vi "Populate Module.vi"(4 "Manifestation Ancestors":T1, 7 "Temporary Template Root Dir":path, 9 "Preloaded Module Class Ref Map":variant, 10 "Module Spec. File":path, 11 "Module LVLib":refnum<vi>) -> (3 "Module LVLib Dup":refnum<vi>)   [LabVIEW 2013]
doc: "Copyright (c) 2016 Sze Howe Koh\n\nThis Source Code Form is subject to the terms of the Mozilla Public License, v. 2.0. If a copy of the MPL was not distributed with this file, You can obtain one at http://mozilla.org/MPL/2.0/."
uses:
  Data Structures/Manifestation Ancestors.ctl
  Param Writers/TypeConv/Category.ctl
  Param Writers/Identity Writer/Identity Writer.lvclass
  Param Writers/Opaque Struct Writer/Opaque Struct Writer.lvclass
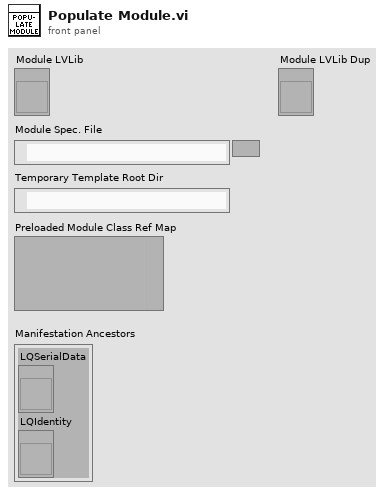
[diagram p1: front panel]
types:
  T1 = typedef "Manifestation Ancestors.ctl" = cluster{"LQSerialData":refnum<vi>, "LQIdentity":refnum<vi>}
  T2 = typedef "Category.ctl" = enum16{"Invalid", "Void", "Boolean", "Numeric", "Enum", "SimpleStruct", "OpaqueStruct", "SimpleIdentity", "QObject", "SimpleContainer", "FullArray"}
  T3 = typedef "Type Categories.ctl" = cluster{"numerics":T4[], "simpleStructs":T5[], "opaqueStructs":T10[], "simpleIdentities":T10[], "qObjects":T10[], "simpleContainers":T4[], "fullArrays":T4[]}
  T4 = typedef "TypeConv.ctl" = cluster{"name":string, "dllType":string}
  T5 = typedef "Simple Struct.ctl" = cluster{"name":string, "fields":T6[], "methods":T7[]}
  T6 = typedef "Param.ctl" = cluster{"name":string, "type":string, "defaultValue":string}
  T7 = typedef "Method.ctl" = cluster{"name":string, "retType":string, "uniqueName":string, "params":T6[], "isConst":bool, "isStaticMember":bool, "isFactory":bool, "connectorPane":T8}
  T8 = typedef "Connector Pane.ctl" = cluster{"pattern":u32, "terminals":T9[]}
  T9 = typedef "Connector Pane Terminal.ctl" = cluster{"name":string, "index":u32}
  T10 = typedef "Class.ctl" = cluster{"name":string, "base":string, "enums":T11[], "methods":T7[], "properties":T13[]}
  T11 = typedef "Enum.ctl" = cluster{"name":string, "values":T12[]}
  T12 = typedef "Enum Value.ctl" = cluster{"name":string, "value":i32}
  T13 = typedef "Property.ctl" = cluster{"name":string, "getter":string, "setter":string}
  T14 = typedef "Namespace.ctl" = cluster{"name":string, "enums":T11[], "methods":T7[]}
  T15 = typedef "Projection Info.ctl" = cluster{"source":string, "projection":string}
  T16 = typedef "LabVIEW Documentation.ctl" = cluster{"classUrlFormat":string, "methodUrlFormat":string}
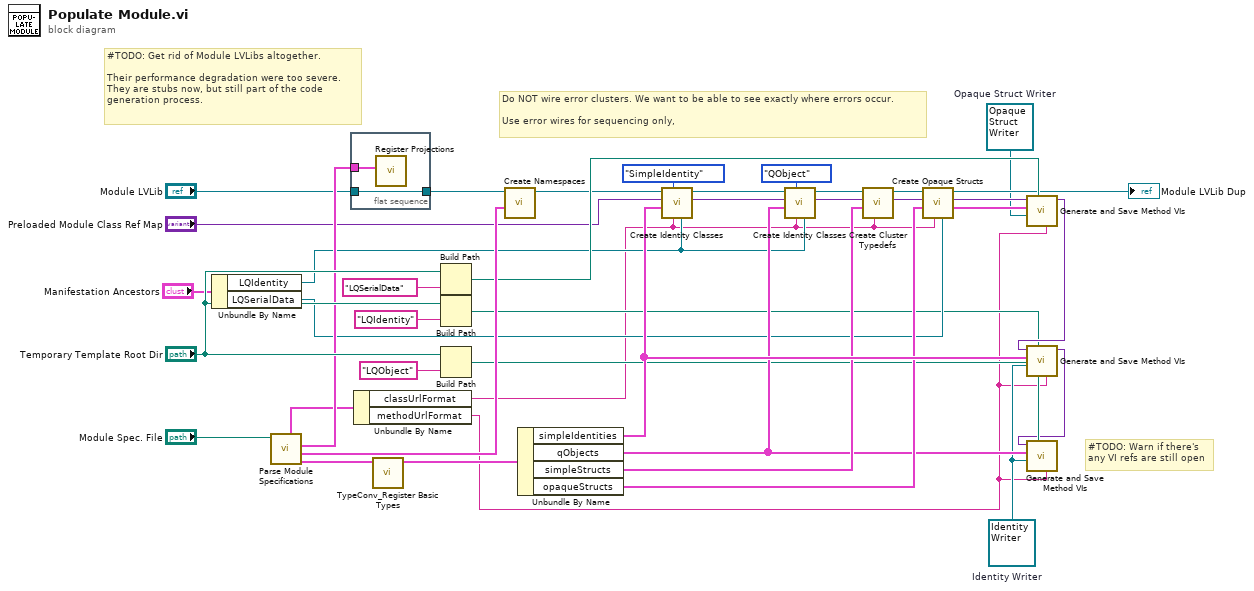
[diagram p0: block diagram]
diagram:
  w8 = refnum<class "Opaque Struct Writer.lvclass"> refnum  # Opaque Struct Writer
  w7 = refnum<class "Identity Writer.lvclass"> refnum  # Identity Writer
  # "#TODO: Get rid of Module LVLibs altogether.\n\nTheir performance degradation were too severe.\nThey are stubs now, but still part of the code\ngeneration process."
  # "#TODO: Warn if there's\nany VI refs are still open"
  # "Do NOT wire error clusters. We want to be able to see exactly where errors occur.\n\nUse error wires for sequencing only,"
  n1 = Unbundle By Name("Manifestation Ancestors") -> ("LQIdentity"=w10:refnum<vi>, "LQSerialData"=w9:refnum<vi>)
  n2 = call "Parse Module Specifications.vi"("Module Spec. File"="Module Spec. File") -> ("Type Categories"=w25:T3, "Namespaces"=w38:T14[], "Projections"=w16:T15[], "LabVIEW Documentation"=w3:T16)  [unwired: 6 in, 1 out]
  n3 = flat-sequence {
    tunnel: w16 -> [w41]
    tunnel: [w40] -> w14
    tunnel: "Module LVLib" -> [w40]
    frame #0 {
      n4 = call "Register Projections.vi"("Projection Info"=w41) -> ()  [unwired: 11 in]
    }
  }
  n5 = Unbundle By Name(w3) -> ("classUrlFormat"=w2:string, "methodUrlFormat"=w1:string)
  n6 = call "TypeConv_Register Basic Types.vi"("Type Categories"=w25) -> ("Type Categories Dup"=w24:T3)  [unwired: 10 in]
  n7 = Build Path(base path="Temporary Template Root Dir", name or relative path="LQSerialData" ("name")) -> (appended path=w26:path)
  n8 = Build Path(base path="Temporary Template Root Dir", name or relative path="LQIdentity" ("name")) -> (appended path=w4:path)
  n9 = Build Path(base path="Temporary Template Root Dir", name or relative path="LQObject" ("name")) -> (appended path=w27:path)
  n10 = call "Create Namespaces.vi"("Namespaces"=w38, "Owning LVLib"=w14) -> ("Owning LVLib Dup"=w23:refnum<vi>)  [unwired: 9 in]
  n11 = Unbundle By Name(w24) -> ("simpleIdentities"=w39:T10[], "qObjects"=w31:T10[], "simpleStructs"=w37:T5[], "opaqueStructs"=w32:T10[])
  n12 = call "Create Identity Classes.vi"("Manifestation Ancestor"=w10, "Class URL Format"=w2, "Category"=Category."SimpleIdentity", "Classes"=w39, "Existing Module Class Ref Map"="Preloaded Module Class Ref Map", "Owning LVLib"=w23) -> ("Augmented Module Class Ref Map"=w18:variant, "Owning LVLib Dup"=w34:refnum<vi>)  [unwired: 4 in]
  n13 = call "Create Identity Classes.vi"("Manifestation Ancestor"=w10, "Class URL Format"=w2, "Category"=Category."QObject", "Classes"=w31, "Existing Module Class Ref Map"=w18, "Owning LVLib"=w34) -> ("Augmented Module Class Ref Map"=w17:variant, "Owning LVLib Dup"=w22:refnum<vi>)  [unwired: 4 in]
  n14 = call "Create Cluster Typedefs.vi"("Struct URL Format"=w2, "Simple Structs"=w37, "Owning LVLib"=w22) -> ("Owning LVLib Dup"=w36:refnum<vi>)  [unwired: 8 in]
  n15 = call "Create Opaque Structs.vi"("Manifestation Ancestor"=w9, "Class URL Format"=w2, "Opaque Structs"=w32, "Existing Class Ref Map"=w17, "Owning LVLib"=w36) -> ("Augmented Class Ref Map"=w12:variant, "Owning LVLib Dup"=→"Module LVLib Dup":refnum<vi>)  [unwired: 5 in]
  n16 = call "Generate and Save Method VIs.vi"("Method URL Format"=w1, "Template VI Dir"=w26, "Class Param Writer"=w8, "Class Info"=w32, "Module Class Ref Map"=w12) -> ("Reduced Module Class Ref Map"=w6:variant)  [unwired: 6 in]
  n17 = call "Generate and Save Method VIs.vi"("Method URL Format"=w1, "Template VI Dir"=w4, "Class Param Writer"=w7, "Class Info"=w39, "Module Class Ref Map"=w6) -> ("Reduced Module Class Ref Map"=w5:variant)  [unwired: 6 in]
  n18 = call "Generate and Save Method VIs.vi"("Method URL Format"=w1, "Template VI Dir"=w27, "Class Param Writer"=w7, "Class Info"=w31, "Module Class Ref Map"=w5) -> ()  [unwired: 6 in, 1 out]
